vi "AMZ_S3_APIHLP_Convert Event String to Enum.vi"(4 "Permission String":string) -> (1 "Event":T1)   [LabVIEW 2015, in "LV Interface for Amazon S3.lvlib"]
doc: "Convert the Permission represented as a String to the Enum typedef representation."
uses:
  LV Interface for Amazon S3.lvlib
  Typedefs/AMZ_S3_Event.ctl
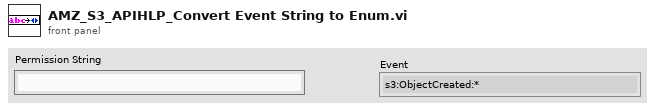
[diagram p1: front panel]
types:
  T1 = typedef "LV Interface for Amazon S3.lvlib/AMZ_S3_Event.ctl" = enum16{"s3:ObjectCreated:*", "s3:ObjectCreated:Put", "s3:ObjectCreated:Post", "s3:ObjectCreated:Copy", "s3:ObjectCreated:CompleteMultipartUpload", "s3:ObjectRemoved:*", "s3:ObjectRemoved:Delete", "s3:ObjectRemoved:DeleteMarkerCreated", "s3:ReducedRedundancyLostObject"}
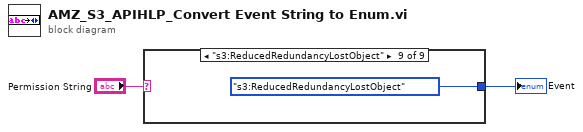
[diagram p0: block diagram]
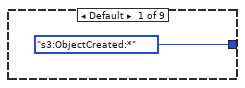
[diagram p2: hidden frame]
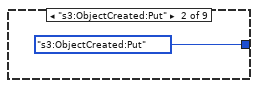
[diagram p3: hidden frame]
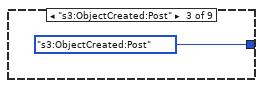
[diagram p4: hidden frame]
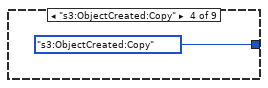
[diagram p5: hidden frame]
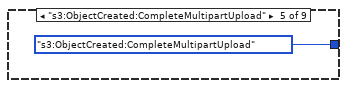
[diagram p6: hidden frame]
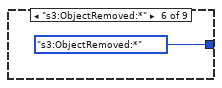
[diagram p7: hidden frame]
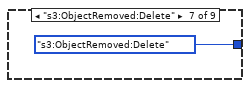
[diagram p8: hidden frame]
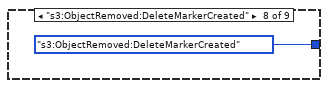
[diagram p9: hidden frame]
diagram:
  n1 = case shown="\"s3:ReducedRedundancyLostObject\"" "Permission String" {
    tunnel: [AMZ_S3_Event."s3:ObjectCreated:*" ("Event") AMZ_S3_Event."s3:ObjectCreated:Put" ("Event") AMZ_S3_Event."s3:ObjectCreated:Post" ("Event") AMZ_S3_Event."s3:ObjectCreated:Copy" ("Event") AMZ_S3_Event."s3:ObjectCreated:CompleteMultipartUpload" ("Event") AMZ_S3_Event."s3:ObjectRemoved:*" ("Event") AMZ_S3_Event."s3:ObjectRemoved:Delete" ("Event") AMZ_S3_Event."s3:ObjectRemoved:DeleteMarkerCreated" ("Event") AMZ_S3_Event."s3:ReducedRedundancyLostObject" ("Event")] -> w1
    frame Default {
    }
    frame "s3:ObjectCreated:Put" {
    }
    frame "s3:ObjectCreated:Post" {
    }
    frame "s3:ObjectCreated:Copy" {
    }
    frame "s3:ObjectCreated:CompleteMultipartUpload" {
    }
    frame "s3:ObjectRemoved:*" {
    }
    frame "s3:ObjectRemoved:Delete" {
    }
    frame "s3:ObjectRemoved:DeleteMarkerCreated" {
    }
    frame "s3:ReducedRedundancyLostObject" {
    }
  }
  "Event" <- w1
